vi "Register gRPC Messages.vi"(8 "error in (no error)":errorcluster, 11 "Template Server in":refnum<class "OCV4.lvclass">) -> (0 "error out":errorcluster, 3 "Template Server out":refnum<class "OCV4.lvclass">)   [LabVIEW 2019, in "OCV4.lvlib" / "OCV4.lvclass"]
uses:
  OCV4.lvclass
  gRPC lvSupport/Server API/typeDefs/Message Metadata.ctl
  gRPC lvSupport/Server API/typeDefs/Message Element Metadata.ctl
  gRPC lvSupport/Server API/typeDefs/Message Element Type.ctl
  OCV4.lvclass/OCV4.ctl
  gRPC lvSupport/gprc-lvsupport.lvlib
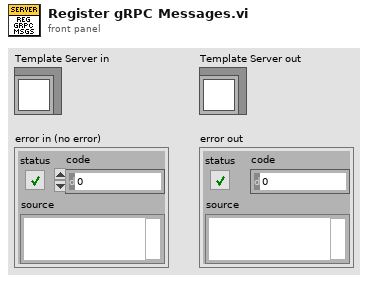
[diagram p1: front panel]
types:
  T1 = typedef "OCV4.lvlib/gprc-lvsupport.lvlib/Message Metadata.ctl" = cluster{"Name":string, "Elements":T2[]}
  T2 = typedef "OCV4.lvlib/gprc-lvsupport.lvlib/Message Element Metadata.ctl" = cluster{"Embedded Message Name":string, "Protobuf Index":i32, "MessageElementType":T3, "Repeated":bool}
  T3 = typedef "OCV4.lvlib/gprc-lvsupport.lvlib/Message Element Type.ctl" = enum32{"Int32Value", "FloatValue", "DoubleValue", "BoolValue", "StringValue", "MessageValue", "Int64Value", "UInt32Value", "UInt64Value", "EnumValue"}
  T4 = typedef "OCV4.lvlib/gprc-lvsupport.lvlib/grpcId.ctl" = u64
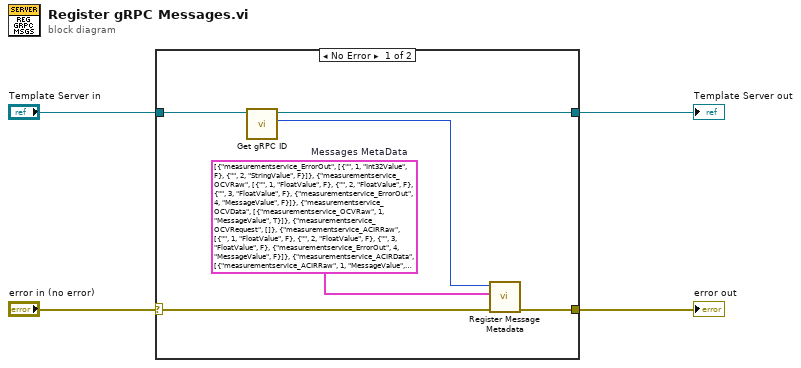
[diagram p0: block diagram]
diagram:
  n1 = case shown="No Error" "error in (no error)" {
    selector: "error in (no error)" -> [w5 w12]
    tunnel: [w10 w11] -> w4
    tunnel: [w9 w12] -> w3
    tunnel: "Template Server in" -> [w7 w11]
    frame No Error {
      w6 = T1[] [{"Name"="measurementservice_ErrorOut", "Elements"=[{"Embedded Message Name"="", "Protobuf Index"=1, "MessageElementType"=enum."Int32Value", "Repeated"=FALSE}, {"Embedded Message Name"="", "Protobuf Index"=2, "MessageElementType"=enum."StringValue", "Repeated"=FALSE}]}, {"Name"="measurementservice_OCVRaw", "Elements"=[{"Embedded Message Name"="", "Protobuf Index"=1, "MessageElementType"=enum."FloatValue", "Repeated"=FALSE}, {"Embedded Message Name"="", "Protobuf Index"=2, "MessageElementType"=enum."FloatValue", "Repeated"=FALSE}, {"Embedded Message Name"="", "Protobuf Index"=3, "MessageElementType"=enum."FloatValue", "Repeated"=FALSE}, {"Embedded Message Name"="measurementservice_ErrorOut", "Protobuf Index"=4, "MessageElementType"=enum."MessageValue", "Repeated"=FALSE}]}, {"Name"="measurementservice_OCVData", "Elements"=[{"Embedded Message Name"="measurementservice_OCVRaw", "Protobuf Index"=1, "MessageElementType"=enum."MessageValue", "Repeated"=TRUE}]}, {"Name"="measurementservice_OCVRequest", "Elements"=[]}, {"Name"="measurementservice_ACIRRaw", "Elements"=[{"Embedded Message Name"="", "Protobuf Index"=1, "MessageElementType"=enum."FloatValue", "Repeated"=FALSE}, {"Embedded Message Name"="", "Protobuf Index"=2, "MessageElementType"=enum."FloatValue", "Repeated"=FALSE}, {"Embedded Message Name"="", "Protobuf Index"=3, "MessageElementType"=enum."FloatValue", "Repeated"=FALSE}, {"Embedded Message Name"="measurementservice_ErrorOut", "Protobuf Index"=4, "MessageElementType"=enum."MessageValue", "Repeated"=FALSE}]}, {"Name"="measurementservice_ACIRData", "Elements"=[{"Embedded Message Name"="measurementservice_ACIRRaw", "Protobuf Index"=1, "MessageElementType"=enum."MessageValue", "Repeated"=TRUE}]}, {"Name"="measurementservice_ACIRRequest", "Elements"=[]}, {"Name"="measurementservice_InvokeRequest", "Elements"=[{"Embedded Message Name"="", "Protobuf Index"=1, "MessageElementType"=enum."StringValue", "Repeated"=FALSE}, {"Embedded Message Name"="", "Protobuf Index"=2, "MessageElementType"=enum."StringValue", "Repeated"=FALSE}]}, {"Name"="measurementservice_InvokeResponse", "Elements"=[{"Embedded Message Name"="", "Protobuf Index"=1, "MessageElementType"=enum."Int32Value", "Repeated"=FALSE}]}, {"Name"="measurementservice_QueryRequest", "Elements"=[{"Embedded Message Name"="", "Protobuf Index"=1, "MessageElementType"=enum."StringValue", "Repeated"=FALSE}]}, {"Name"="measurementservice_QueryResponse", "Elements"=[{"Embedded Message Name"="", "Protobuf Index"=1, "MessageElementType"=enum."StringValue", "Repeated"=FALSE}, {"Embedded Message Name"="", "Protobuf Index"=2, "MessageElementType"=enum."Int32Value", "Repeated"=FALSE}]}, {"Name"="measurementservice_RegistrationRequest", "Elements"=[{"Embedded Message Name"="", "Protobuf Index"=1, "MessageElementType"=enum."StringValue", "Repeated"=FALSE}]}, {"Name"="measurementservice_ServerEvent", "Elements"=[{"Embedded Message Name"="", "Protobuf Index"=1, "MessageElementType"=enum."StringValue", "Repeated"=FALSE}, {"Embedded Message Name"="", "Protobuf Index"=2, "MessageElementType"=enum."Int32Value", "Repeated"=FALSE}, {"Embedded Message Name"="", "Protobuf Index"=3, "MessageElementType"=enum."Int32Value", "Repeated"=FALSE}]}]  # Messages MetaData
      n2 = call "Get gRPC ID.vi"("OOP Server in"=w7) -> ("gRPC ID"=w8:T4, "OOP Server out"=w10:refnum<class "OCV4.lvclass">)  [unwired: 9 in]
      n3 = call "Register Message Metadata.vi"("error in (no error)"=w5, "Messages"=w6, "gRPCid"=w8) -> ("error out"=w9:errorcluster)  [unwired: 7 in, 1 out]
    }
    frame Error {
    }
  }
  "Template Server out" <- w4
  "error out" <- w3
